vi "Write.vi"(6 "Append Index":i32, 8 "error in (no error)":errorcluster, 9 "Notes":string, 10 "Data (Dictionary)":T1[](array[typedef]), 11 "Data.S3":refnum<class "LV-Data.S3.lvclass">) -> (0 "error out":errorcluster, 3 "Data.S3 out":refnum<class "LV-Data.S3.lvclass">, 5 "Path out":path)   [LabVIEW 2019, in "LV-Data.S3.lvclass"]
uses:
  LV-Data.S3.lvclass
  LV-Data/Typedefs/Dictionary--cluster.ctl
  LV-Data/LV-Data.lvclass
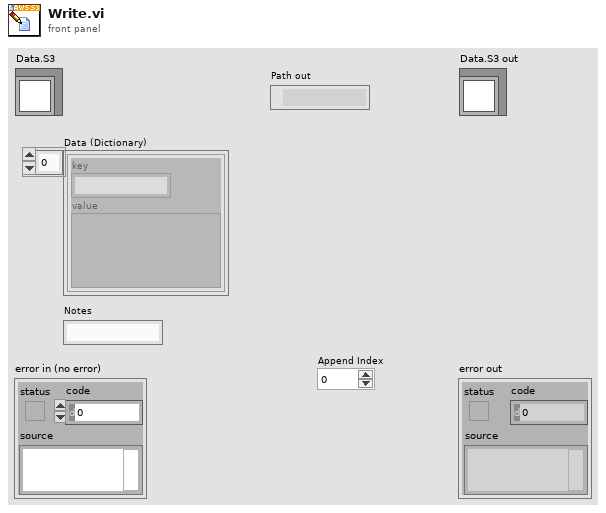
[diagram p1: front panel]
types:
  T1 = typedef "LV-Data.lvclass/Dictionary--cluster.ctl" = cluster{"key":string, "value":variant}
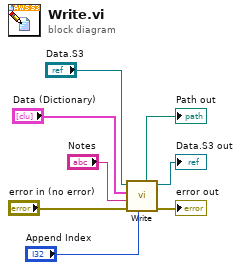
[diagram p0: block diagram]
diagram:
  n1 = call-parent "Write.vi"("Append Index"="Append Index", "error in (no error)"="error in (no error)", "Notes"="Notes", "Data (Dictionary)"="Data (Dictionary)", "Data in"="Data.S3") -> ("error out"=→"error out":errorcluster, "Data out"=→"Data.S3 out":refnum<class "LV-Data.S3.lvclass">, "Path out"=→"Path out":path)  [unwired: 4 in]
